vi "GlobalExposure.vi"() -> ()   [LabVIEW 2010]
panel:
  in  "Exposure":dbl format="%.2f"
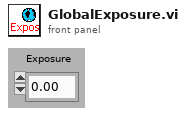
[diagram p1: front panel]
diagram:
